vi "Flip Image.vi"(7 "Direction":T1, 8 "error in (no error)":errorcluster, 11 "Image":T2) -> (0 "error out":errorcluster, 3 "Flipped Image":T2)   [LabVIEW 2020, in "G-Image.lvlib"]
doc: "Flips the image horizontally or vertically."
uses:
  G-Image.lvlib
  <vilib>/picture/picture.llb/imagedata.ctl
  Controls/Flip Direction.ctl
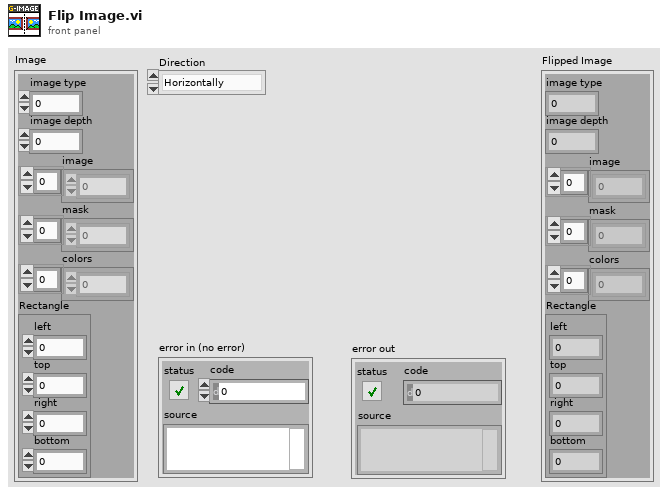
[diagram p1: front panel]
types:
  T1 = typedef "G-Image.lvlib/Flip Direction.ctl" = enum16{"Horizontally", "Vertically"}
  T2 = typedef "imagedata.ctl" = cluster{"image type":i32, "image depth":i32, "image":u8[], "mask":u8[], "colors":u32[], "Rectangle":cluster{"left":i16, "top":i16, "right":i16, "bottom":i16}}
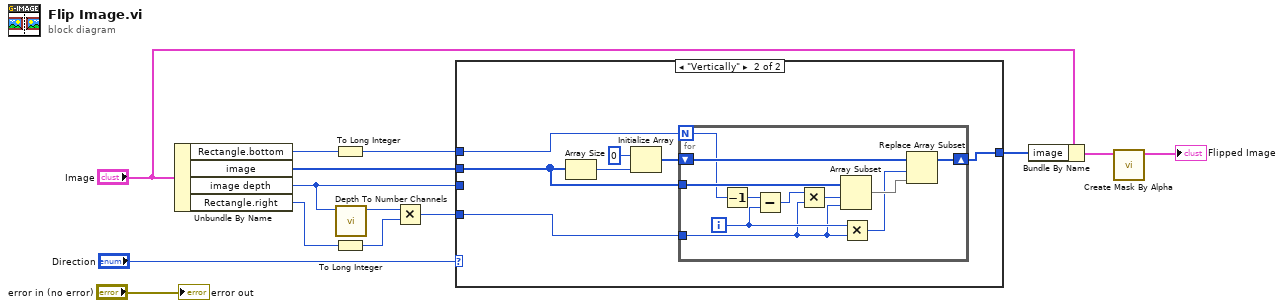
[diagram p0: block diagram]
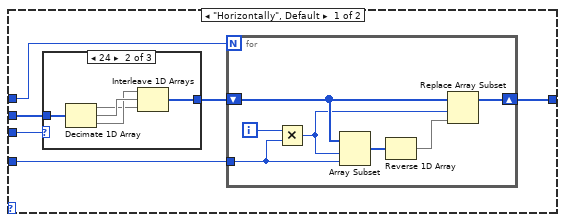
[diagram p2: hidden frame]
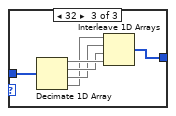
[diagram p4: hidden frame]
diagram:
  n1 = Unbundle By Name("Image") -> ("Rectangle.bottom"=w9:i16, "image"=w10:u8[], "image depth"=w1:i32, "Rectangle.right"=w3:i16)
  n2 = To Long Integer(number=w9) -> (32bit integer=w8:i32)
  n3 = To Long Integer(number=w3) -> (32bit integer=w2:i32)
  n4 = call "Depth To Number Channels.vi"("Depth"=w1) -> ("Channels"=w5:i32)  [unwired: 10 in]
  n5 = Multiply(x=w5, y=w2) -> (x*y=w4:i32)
  n6 = case shown="\"Vertically\"" "Direction" {
    tunnel: [w20 w41] -> w12
    tunnel: w10 -> [w19 w42]
    tunnel: w1 -> [w18 _]
    tunnel: w8 -> [w16 w43]
    tunnel: w4 -> [w15 w40]
    frame "Horizontally", Default {
      n7 = case shown="24" w18 {
        tunnel: [w21 w26 w32] -> w17
        tunnel: w19 -> [w21 w25 w31]
        frame 0, Default {
        }
        frame 24 {
          n8 = Decimate 1D Array(w25) -> (w22:u8[], w24:u8[], w23:u8[])
          n9 = Interleave 1D Arrays(w23, w24, w22) -> (w26:u8[])
        }
        frame 32 {
          n10 = Decimate 1D Array(w31) -> (w30:u8[], w29:u8[], w28:u8[], w27:u8[])
          n11 = Interleave 1D Arrays(w27, w28, w29, w30) -> (w32:u8[])
        }
      }
      n12 = for {
        N: w16 -> [_]
        shift-right: [w33] -> w20
        shift-left: w17 -> [w37]
        tunnel: w15 -> [w38]
        i -> [w39]
        n13 = Multiply(x=w39, y=w38) -> (x*y=w34:i32)
        n14 = Array Subset(array=w37, index=w34, length=w38) -> (w36:u8[])
        n15 = Reverse 1D Array(array=w36) -> (reversed array=w35:u8[])
        n16 = Replace Array Subset(array=w37, new element=w35, index=w34) -> (w33:u8[])
      }
    }
    frame "Vertically" {
      n17 = Array Size(array=w42) -> (size(s)=w44:i32)
      n18 = Initialize Array(u8 0, w44) -> (w46:u8[])
      n19 = for {
        N: w43 -> [w53]
        shift-right: [w55] -> w41
        shift-left: w46 -> [w56]
        tunnel: w42 -> [w57]
        tunnel: w40 -> [w47]
        i -> [w52]
        n20 = Decrement(x=w53) -> (x-1=w51:i32)
        n21 = Subtract(x=w51, y=w52) -> (x-y=w50:i32)
        n22 = Multiply(x=w50, y=w47) -> (x*y=w48:i32)
        n23 = Array Subset(array=w57, index=w48, length=w47) -> (w54:u8[])
        n24 = Multiply(x=w52, y=w47) -> (x*y=w49:i32)
        n25 = Replace Array Subset(array=w56, new element=w54, index=w49) -> (w55:u8[])
      }
    }
  }
  n26 = Bundle By Name(cluster="Image", "image"=w12) -> (w11:T2)
  n27 = call <vilib>:"Create Mask By Alpha.vi"("image data"=w11) -> ("masked image data"=→"Flipped Image":T2)  [unwired: 10 in]
  "error out" <- "error in (no error)"
